vi "Blocking Read Before Fulfill.vi"(8 "error in (no error)":errorcluster) -> (0 "error out":errorcluster)   [LabVIEW 2017, in "Unit Tests.lvlib"]
uses:
  Unit Tests.lvlib
  675f34c3-de2a-4eca-afed-97da1a23b3ea.vi
  f4ded3e2-5877-4285-a1a8-ead4dd134e79.vi
  4e1b5ce0-e1b8-49ea-b8a3-943737b07833.vi
  Promise Future/Promise/Promise.lvclass
  E:/Promise/Promise Future/Future/Future.lvclass
  Promise Future/Promise/Read Future.vi
  Promise Future/Future/Read Value.vi
  Promise Future/Future/Write Future.vi
  Promise Future/Future/Future.lvclass
  <vilib>/addons/_JKI Toolkits/Caraya/classes/Test/Test.lvclass
  <vilib>/addons/_JKI Toolkits/Caraya/classes/Assert/Assert.lvclass
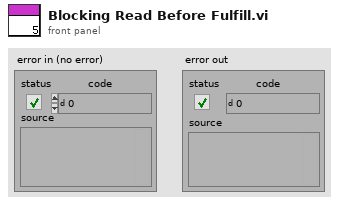
[diagram p1: front panel]
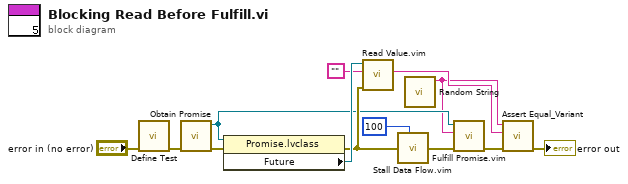
[diagram p0: block diagram]
diagram:
  n1 = call <vilib>:"Define Test.vi"("error in (no error)"="error in (no error)") -> ("error out"=w6:errorcluster)  [unwired: 10 in]
  n2 = call "Obtain Promise.vi"("error in (no error)"=w6) -> ("error out"=w13:errorcluster, "Promise out"=w5:refnum<class "Promise.lvclass">)  [unwired: 8 in, 1 out]
  n3 = property class="Promise.lvclass"(reference=w5, error in=w13) -> (error out=w11:errorcluster, "Future"=w12:refnum<class "Future.lvclass">)  [unwired: 1 out]
  n4 = call "Read Value.vim"("error in (no error)"=w11, "Default Value"="", "Future in"=w12) -> ("Value"=w2:string)  [unwired: 5 in, 3 out]
  n5 = call "Stall Data Flow.vim"("value in"=w11, "milliseconds to wait"=u32 100) -> ("value out"=w8:errorcluster)  [unwired: 1 out]
  n6 = call "Random String.vi"() -> ("string"=w1:string)  [unwired: 11 in]
  n7 = call "Fulfill Promise.vim"("error in (no error)"=w8, "Value"=w1, "Promise in"=w5) -> ("error out"=w4:errorcluster)  [unwired: 7 in, 1 out]
  n8 = call <vilib>:"Assert Equal_Variant.vi"("error in (no error)"=w4, "Y"=w2, "X"=w1) -> ("error out"=→"error out":errorcluster)  [unwired: 8 in]
